vi "I8_to_String.vi"(5 "number":i8, 6 "error in (no error)":errorcluster, 9 "string in":string) -> (0 "error out":errorcluster, 3 "String Out":string)   [LabVIEW 2015, in "Ion Motion Roboclaw.lvlib"]
uses:
  <instrlib>/Ion Motion Roboclaw/Ion Motion Roboclaw.lvlib
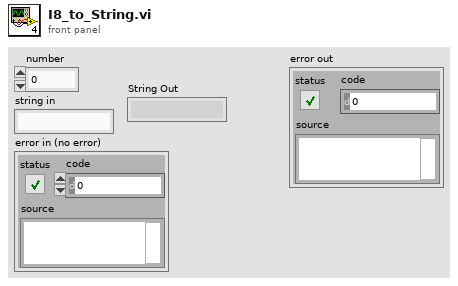
[diagram p1: front panel]
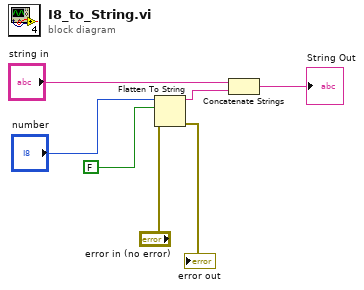
[diagram p0: block diagram]
diagram:
  n1 = Flatten To String(anything="number", prepend array or string size? (T)=FALSE, error in (no error)="error in (no error)") -> (data string=w4:string, error out=→"error out":errorcluster)  [unwired: 1 in, 1 out]
  n2 = Concatenate Strings("string in", w4) -> (→"String Out":string)
